vi "Encoder Begin.vi"() -> (0 "error out":errorcluster)   [LabVIEW 2012]
uses:
  <vilib>/Rock Robotics/SystemInterfaces/DIO/FPGA_DIOChannel.ctl
  <vilib>/Rock Robotics/WPI/Encoder/WPI_EncoderType.ctl
  <vilib>/Rock Robotics/WPI/Counter/WPI_CounterDigitalInputToDigitalSource.vi
  <vilib>/Rock Robotics/WPI/Counter/WPI_CounterOpen UpDown Mode.vi
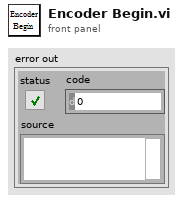
[diagram p1: front panel]
types:
  T1 = typedef "FPGA_DIOChannel.ctl" = enum8{"DIO 1", "DIO 2", "DIO 3", "DIO 4", "DIO 5", "DIO 6", "DIO 7", "DIO 8", "DIO 9", "DIO 10", "DIO 11", "DIO 12", "DIO 13", "DIO 14", "Invalid"}
  T2 = typedef "WPI_EncoderType.ctl" = enum16{"1x", "2x", "4x"}
  T3 = typedef "WPI_DigitalInputDevRef.ctl" = cluster{"DevStatus":errorcluster, "DIO Channel":T1, "Digital Module":T4}
  T4 = typedef "FPGA_TypedefDigitalModule.ctl" = enum16{"Digital Module 1", "Digital Module 2"}
  T5 = typedef "FPGA_CounterEncoderSourceConvertionLVSourceType.ctl" = cluster{"DevStatus":errorcluster, "AnalogTriggerMode?":bool, "DigitalMode":cluster{"Digital Module":T4, "DIO Channel":T6}, "AnalogTriggerMode":cluster{"AnalogTriggerIndex":T7, "OutputType":T8}}
  T6 = typedef "FPGA_DIODigitalSourceChannel.ctl" = enum8{"DIO 1", "DIO 2", "DIO 3", "DIO 4", "DIO 5", "DIO 6", "DIO 7", "DIO 8", "DIO 9", "DIO 10", "DIO 11", "DIO 12", "DIO 13", "DIO 14", "Disabled"}
  T7 = typedef "FPGA_AnalogTriggerIndex.ctl" = enum8{"Trig 0", "Trig 1", "Trig 2", "Trig 3", "Trig 4", "Trig 5", "Trig 6", "Trig 7", "Invalid"}
  T8 = typedef "FPGA_AnalogTriggerOutType.ctl" = enum16{"InWindow", "TriggerState", "Rising", "Falling"}
  T9 = typedef "WPI_CounterDevRef.ctl" = cluster{"DevStatus":errorcluster, "CntIndex":T10}
  T10 = typedef "FPGA_CounterCtrSystemIndex.ctl" = enum8{"Ctr 0", "Ctr 1", "Ctr 2", "Ctr 3", "Ctr 4", "Ctr 5", "Ctr 6", "Ctr 7", "Invalid"}
  T11 = typedef "WPI_EncoderDevRef.ctl" = cluster{"DevStatus":errorcluster, "EncoderIndex":T12, "CounterIndex":T10, "DistancePerCount":dbl, "Decoding Type":T2}
  T12 = typedef "FPGA_EncoderIdx.ctl" = enum8{"Enc 0", "Enc 1", "Enc 2", "Enc 3", "Invalid"}
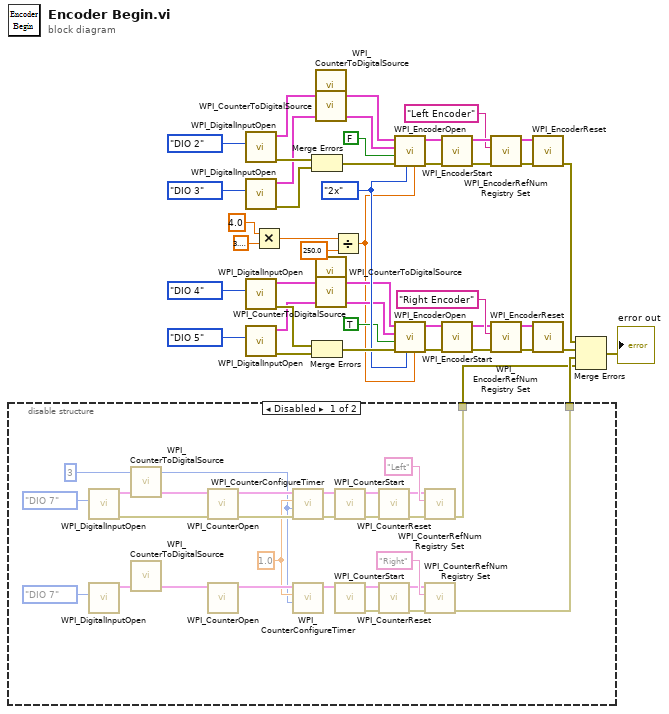
[diagram p0: block diagram]
diagram:
  w35 = WPI_EncoderType."2x" ("Decoding Type")
  n1 = disable-structure shown="Disabled" {
    disable-tunnel: [w49 _] -> w2
    disable-tunnel: [w48 _] -> w1
    frame Disabled {
      w46 = u8 3 ("Number Samples to Average")
      w47 = 1.0 ("MaxPeriod (sec)")
      n2 = call <vilib>:"WPI_DigitalInputOpen.vi"("DIO Channel"=FPGA_DIOChannel."DIO 7") -> ("error out"=w54:errorcluster, "DigitalInputDevRef"=w65:T3)  [unwired: 9 in]
      n3 = call <vilib>:"WPI_DigitalInputOpen.vi"("DIO Channel"=FPGA_DIOChannel."DIO 7") -> ("DigitalInputDevRef"=w71:T3)  [unwired: 9 in, 1 out]
      n4 = call-poly <vilib>:"WPI_CounterToDigitalSource.vi"("DigitalInputDevRef"=w65) -> ("Digital Source"=w64:T5)  [unwired: 6 in]
      n5 = call-poly <vilib>:"WPI_CounterToDigitalSource.vi"("DigitalInputDevRef"=w71) -> ("Digital Source"=w70:T5)  [unwired: 6 in]
      n6 = call-poly <vilib>:"WPI_CounterOpen.vi"("error in (no error)"=w54, "Up Source"=w64) -> ("error out"=w55:errorcluster, "CounterDevRef"=w63:T9)  [unwired: 8 in]
      n7 = call-poly <vilib>:"WPI_CounterOpen.vi"("Up Source"=w70) -> ("CounterDevRef"=w69:T9)  [unwired: 9 in, 1 out]
      n8 = call <vilib>:"WPI_CounterConfigureTimer.vi"("error in (no error)"=w55, "Number Samples to Average"=w46, "MaxPeriod (sec)"=w47, "CounterDevRef in"=w63) -> ("error out"=w56:errorcluster, "CounterDevRef out"=w62:T9)  [unwired: 6 in]
      n9 = call <vilib>:"WPI_CounterConfigureTimer.vi"("Number Samples to Average"=w46, "MaxPeriod (sec)"=w47, "CounterDevRef in"=w69) -> ("CounterDevRef out"=w68:T9)  [unwired: 7 in, 1 out]
      n10 = call <vilib>:"WPI_CounterStart.vi"("error in (no error)"=w56, "CounterDevRef in"=w62) -> ("error out"=w57:errorcluster, "CounterDevRef out"=w58:T9)  [unwired: 8 in]
      n11 = call <vilib>:"WPI_CounterStart.vi"("CounterDevRef in"=w68) -> ("error out"=w59:errorcluster, "CounterDevRef out"=w60:T9)  [unwired: 9 in]
      n12 = call <vilib>:"WPI_CounterReset.vi"("error in (no error)"=w57, "CounterDevRef in"=w58) -> ("error out"=w53:errorcluster, "CounterDevRef out"=w52:T9)  [unwired: 8 in]
      n13 = call <vilib>:"WPI_CounterReset.vi"("error in (no error)"=w59, "CounterDevRef in"=w60) -> ("error out"=w51:errorcluster, "CounterDevRef out"=w50:T9)  [unwired: 8 in]
      n14 = call <vilib>:"WPI_CounterRefNum Registry Set.vi"("error in (no error)"=w53, "refnum name"="Left", "CounterDevRef"=w52) -> ("error out"=w48:errorcluster)  [unwired: 7 in, 1 out]
      n15 = call <vilib>:"WPI_CounterRefNum Registry Set.vi"("error in (no error)"=w51, "refnum name"="Right", "CounterDevRef"=w50) -> ("error out"=w49:errorcluster)  [unwired: 7 in, 1 out]
    }
    frame Enabled {
    }
  }
  n16 = call <vilib>:"WPI_DigitalInputOpen.vi"("DIO Channel"=FPGA_DIOChannel."DIO 2") -> ("error out"=w39:errorcluster, "DigitalInputDevRef"=w20:T3)  [unwired: 9 in]
  n17 = call <vilib>:"WPI_DigitalInputOpen.vi"("DIO Channel"=FPGA_DIOChannel."DIO 3") -> ("error out"=w40:errorcluster, "DigitalInputDevRef"=w18:T3)  [unwired: 9 in]
  n18 = call <vilib>:"WPI_DigitalInputOpen.vi"("DIO Channel"=FPGA_DIOChannel."DIO 4") -> ("error out"=w36:errorcluster, "DigitalInputDevRef"=w29:T3)  [unwired: 9 in]
  n19 = call <vilib>:"WPI_DigitalInputOpen.vi"("DIO Channel"=FPGA_DIOChannel."DIO 5") -> ("error out"=w37:errorcluster, "DigitalInputDevRef"=w27:T3)  [unwired: 9 in]
  n20 = Multiply(x=4.0 ("DistancePerCount"), y=3.141592653589793) -> (x*y=w6:dbl)
  n21 = Merge Errors(w39, w40) -> (w41:errorcluster)
  n22 = Merge Errors(w36, w37) -> (w38:errorcluster)
  n23 = call-poly <vilib>:"WPI_CounterToDigitalSource.vi"("DigitalInputDevRef"=w20) -> ("Digital Source"=w16:T5)  [unwired: 6 in]
  n24 = call-poly <vilib>:"WPI_CounterToDigitalSource.vi"("DigitalInputDevRef"=w18) -> ("Digital Source"=w15:T5)  [unwired: 6 in]
  n25 = call-poly <vilib>:"WPI_CounterToDigitalSource.vi"("DigitalInputDevRef"=w29) -> ("Digital Source"=w25:T5)  [unwired: 6 in]
  n26 = call-poly <vilib>:"WPI_CounterToDigitalSource.vi"("DigitalInputDevRef"=w27) -> ("Digital Source"=w24:T5)  [unwired: 6 in]
  n27 = Divide(x=w6, y=250.0) -> (x/y=w3:dbl)
  n28 = call <vilib>:"WPI_EncoderOpen.vi"("DistancePerCount"=w3, "Decoding Type"=w35, "error in (no error)"=w41, "Invert Direction (False)"=FALSE, "BSource"=w15, "ASource"=w16) -> ("error out"=w43:errorcluster, "EncoderDevRef"=w42:T11)  [unwired: 4 in]
  n29 = call <vilib>:"WPI_EncoderOpen.vi"("DistancePerCount"=w3, "Decoding Type"=w35, "error in (no error)"=w38, "Invert Direction (False)"=TRUE, "BSource"=w24, "ASource"=w25) -> ("error out"=w45:errorcluster, "EncoderDevRef"=w44:T11)  [unwired: 4 in]
  n30 = call <vilib>:"WPI_EncoderStart.vi"("error in (no error)"=w43, "EncoderDevRef"=w42) -> ("error out"=w23:errorcluster, "EncoderDevRef"=w22:T11)  [unwired: 8 in]
  n31 = call <vilib>:"WPI_EncoderStart.vi"("error in (no error)"=w45, "EncoderDevRef"=w44) -> ("error out"=w31:errorcluster, "EncoderDevRef"=w30:T11)  [unwired: 8 in]
  n32 = call <vilib>:"WPI_EncoderRefNum Registry Set.vi"("error in (no error)"=w23, "refnum name"="Left Encoder", "EncoderDevRef"=w22) -> ("error out"=w13:errorcluster, "EncoderDevRef"=w12:T11)  [unwired: 7 in]
  n33 = call <vilib>:"WPI_EncoderRefNum Registry Set.vi"("error in (no error)"=w31, "refnum name"="Right Encoder", "EncoderDevRef"=w30) -> ("error out"=w10:errorcluster, "EncoderDevRef"=w11:T11)  [unwired: 7 in]
  n34 = call <vilib>:"WPI_EncoderReset.vi"("error in (no error)"=w13, "EncoderDevRef"=w12) -> ("error out"=w8:errorcluster)  [unwired: 8 in, 1 out]
  n35 = call <vilib>:"WPI_EncoderReset.vi"("error in (no error)"=w10, "EncoderDevRef"=w11) -> ("error out"=w9:errorcluster)  [unwired: 8 in, 1 out]
  n36 = Merge Errors(w8, w9, w2, w1) -> (→"error out":errorcluster)
